vi "Corr Digitizer Save INFO raw.vi"(7 "path template":path, 8 "error in":errorcluster, 9 "digitizer info":T2, 10 "correction type":T1, 11 "path result":path) -> (0 "error out":errorcluster)   [LabVIEW 2020]
doc: "Saves digitizer/channel INFO file."
uses:
  Corr Digitizer INFO.ctl
  Corr Digitizer INFO item.ctl
  Corr Digitizer INFO parameter.ctl
  Corr CSV Template.ctl
  Corr Digitizer Type.ctl
  octave/infolib/String.vi
  octave/infolib/1D String.vi
  octave/infolib/I64.vi
  octave/infolib/2D String.vi
  octave/infolib/infolib.lvlib
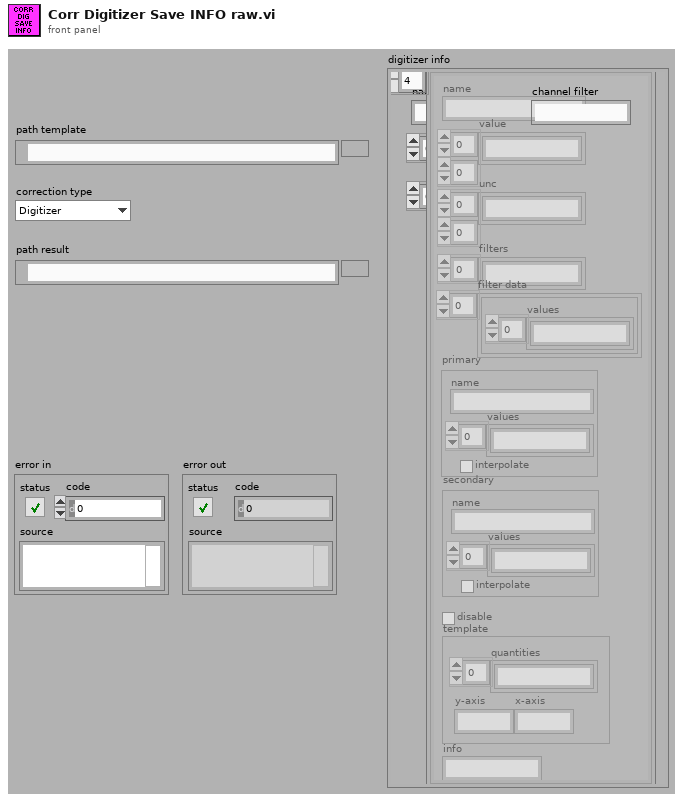
[diagram p1: front panel]
types:
  T1 = typedef "Corr Digitizer Type.ctl" = enum16{"Digitizer", "Channel"}
  T2 = typedef "Corr Digitizer INFO.ctl" = cluster{"name":string, "identifiers":string[], "channel files":string[], "items":T3[], "channel filter":string}
  T3 = typedef "Corr Digitizer INFO item.ctl" = cluster{"name":string, "value":string[][], "unc":string[][], "filters":string[], "primary":T4, "secondary":T4, "filter data":cluster{"values":string[]}[], "disable":bool, "template":T5, "info":string}
  T4 = typedef "Corr Digitizer INFO parameter.ctl" = cluster{"values":string[], "interpolate":bool, "name":string}
  T5 = typedef "Corr CSV Template.ctl" = cluster{"quantities":string[], "y-axis":string, "x-axis":string}
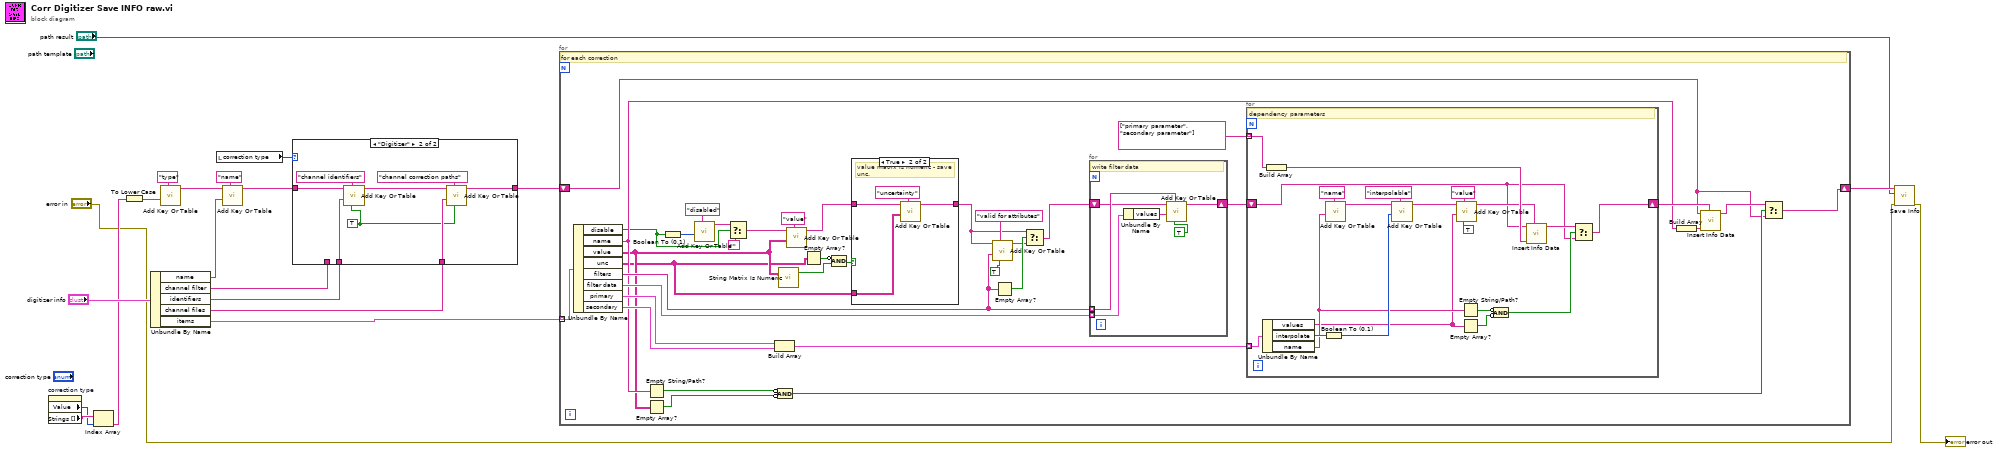
[diagram p0: block diagram]
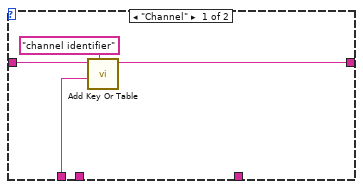
[diagram p3: hidden frame]
diagram:
  n1 = property on="correction type" class="Enum (strict)"() -> ("Value"=w19:T1, "Strings []"=w20:string[])  [unwired: 2 in, 2 out]
  n2 = Index Array(array=w20, index=w19) -> (element=w8:string)
  n3 = To Lower Case(string=w8) -> (all lower case string=w3:string)
  n4 = Unbundle By Name("digitizer info") -> ("name"=w15:string, "channel filter"=w14:string, "identifiers"=w12:string[], "channel files"=w11:string[], "items"=w10:T3[])
  n5 = call-poly "Add Key Or Table.vi"("key description"="type", "string"=w3) -> ("info data out"=w2:string)  [unwired: 8 in, 1 out]
  n6 = local read "correction type"() -> (w13:T1)
  n7 = call-poly "Add Key Or Table.vi"("key description"="name", "string"=w15, "info data"=w2) -> ("info data out"=w1:string)  [unwired: 7 in, 1 out]
  n8 = case shown="\"Digitizer\"" w13 {
    tunnel: w1 -> [w22 w28]
    tunnel: w14 -> [w23 _]
    tunnel: [w21 w26] -> w9
    tunnel: w12 -> [_ w31]
    tunnel: w11 -> [_ w29]
    frame "Channel" {
      n9 = call-poly "Add Key Or Table.vi"("key description"="channel identifier", "string"=w23, "info data"=w22) -> ("info data out"=w21:string)  [unwired: 7 in, 1 out]
    }
    frame "Digitizer" {
      w25 = TRUE ("column vector (F)")
      n10 = call-poly "Add Key Or Table.vi"("collumn vector (F)"=w25, "key description"="channel identifiers", "string"=w31, "info data"=w28) -> ("info data out"=w27:string)  [unwired: 6 in, 1 out]
      n11 = call-poly "Add Key Or Table.vi"("collumn vector (F)"=w25, "key description"="channel correction paths", "string"=w29, "info data"=w27) -> ("info data out"=w26:string)  [unwired: 6 in, 1 out]
    }
  }
  n12 = for {
    tunnel: w10 -> [w68] mode=indexing
    shift-right: [w41] -> w7
    shift-left: w9 -> [w39]
    # "for each correction"
    n13 = Unbundle By Name(w68) -> ("disable"=w48:bool, "name"=w53:string, "value"=w37:string[][], "unc"=w34:string[][], "filters"=w62:string[], "filter data"=w63:cluster{"values":string[]}[], "primary"=w60:T4, "secondary"=w59:T4)
    n14 = Empty String/Path?(string/path=w53) -> (empty?=w57:bool)
    n15 = Empty Array?(array=w37) -> (empty?=w56:bool)
    n16 = Boolean To (0,1)(Boolean=w48) -> (0, 1=w50:i16)
    n17 = call-poly "Add Key Or Table.vi"("key description"="disabled" ("key description to replace"), "numeric"=w50) -> ("info data out"=w47:string)  [unwired: 8 in, 1 out]
    n18 = Select(t=w47, s=w48, f="") -> (s? t:f=w45:string)
    n19 = Build Array(w60, w59) -> (w58:T4[])
    n20 = Compound Arithmetic op=AND(invert w57, invert w56) -> (w55:bool)
    n21 = call "String Matrix Is Numeric.vi"("string matrix"=w37) -> ("is numeric"=w36:bool)  [unwired: 1 in, 1 out]
    n22 = call-poly "Add Key Or Table.vi"("key description"="value", "string"=w37, "info data"=w45) -> ("info data out"=w44:string)  [unwired: 7 in, 1 out]
    n23 = Empty Array?(array=w34) -> (empty?=w38:bool)
    n24 = Compound Arithmetic op=AND(invert w38, w36) -> (w35:bool)
    n25 = case shown="True" w35 {
      tunnel: w44 -> [w95 w97]
      tunnel: w34 -> [_ w98]
      tunnel: [w95 w96] -> w43
      frame False {
        # "value is text - no uncertainty\ndata are CSV files"
      }
      frame True {
        # "value matrix is numeric - save unc."
        n26 = call-poly "Add Key Or Table.vi"("key description"="uncertainty", "string"=w98, "info data"=w97) -> ("info data out"=w96:string)  [unwired: 7 in, 1 out]
      }
    }
    n27 = call-poly "Add Key Or Table.vi"("collumn vector (F)"=TRUE ("column vector (F)"), "key description"="valid for attributes", "string"=w62, "info data"=w43) -> ("info data out"=w64:string)  [unwired: 6 in, 1 out]
    n28 = Empty Array?(array=w62) -> (empty?=w65:bool)
    n29 = Select(t=w43, s=w65, f=w64) -> (s? t:f=w42:string)
    n30 = for {
      tunnel: w63 -> [w94] mode=indexing
      shift-right: [w90] -> w40
      shift-left: w42 -> [w91]
      tunnel: w62 -> [w93] mode=indexing
      # "write filter data"
      n31 = Unbundle By Name(w94) -> ("values"=w92:string[])
      n32 = call-poly "Add Key Or Table.vi"("collumn vector (F)"=TRUE ("column vector (F)"), "key description"=w93, "string"=w92, "info data"=w91) -> ("info data out"=w90:string)  [unwired: 6 in, 1 out]
    }
    n33 = for {
      tunnel: string[] ["primary parameter", "secondary parameter"] -> [w77] mode=indexing
      tunnel: w58 -> [w87] mode=indexing
      shift-right: [w70] -> w54
      shift-left: w40 -> [w71]
      # "dependency parameters"
      n34 = Unbundle By Name(w87) -> ("values"=w81:string[], "interpolate"=w85:bool, "name"=w82:string)
      n35 = Build Array(w77) -> (w76:string[])
      n36 = Boolean To (0,1)(Boolean=w85) -> (0, 1=w84:i16)
      n37 = call-poly "Add Key Or Table.vi"("key description"="name", "string"=w82) -> ("info data out"=w74:string)  [unwired: 8 in, 1 out]
      n38 = call-poly "Add Key Or Table.vi"("key description"="interpolable", "numeric"=w84, "info data"=w74) -> ("info data out"=w73:string)  [unwired: 7 in, 1 out]
      n39 = call-poly "Add Key Or Table.vi"("collumn vector (F)"=TRUE ("column vector (F)"), "key description"="value", "string"=w81, "info data"=w73) -> ("info data out"=w72:string)  [unwired: 6 in, 1 out]
      n40 = Empty String/Path?(string/path=w82) -> (empty?=w80:bool)
      n41 = Empty Array?(array=w81) -> (empty?=w79:bool)
      n42 = Compound Arithmetic op=AND(invert w80, invert w79) -> (w78:bool)
      n43 = call "Insert Info Data.vi"("info data to insert"=w72, "sections"=w76, "info data"=w71) -> ("info data out"=w75:string)  [unwired: 7 in, 1 out]
      n44 = Select(t=w75, s=w78, f=w71) -> (s? t:f=w70:string)
    }
    n45 = Build Array(w53) -> (w52:string[])
    n46 = call "Insert Info Data.vi"("info data to insert"=w54, "sections"=w52, "info data"=w39) -> ("info data out"=w51:string)  [unwired: 7 in, 1 out]
    n47 = Select(t=w51, s=w55, f=w39) -> (s? t:f=w41:string)
  }
  n48 = call "Save Info.vi"("error in"="error in", "filename"="path result", "info data"=w7) -> ("error out"=→"error out":errorcluster)  [unwired: 8 in]
